vi "题目2.vi"() -> ()   [LabVIEW 2017]
uses:
  <vilib>/Waveform/WDTFileIO.llb/ Write Waveform to File.vi
  <vilib>/Waveform/WDTFileIO.llb/Read Waveform from File.vi
  <vilib>/measure/NI_MABase.lvlib
panel:
  out "first waveform in record":waveform(dbl) caption="记录中第一波形"
  out "波形图":waveform(dbl)(graph)
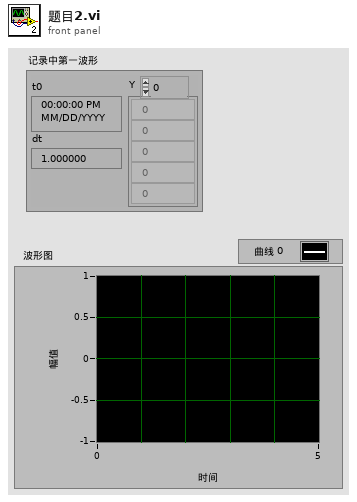
[diagram p1: front panel]
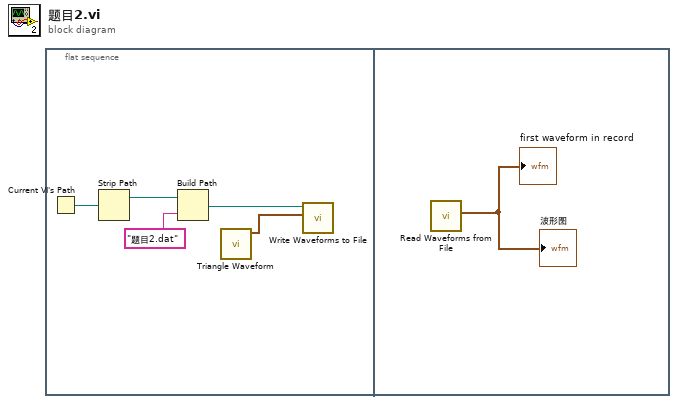
[diagram p0: block diagram]
diagram:
  n1 = flat-sequence {
    frame #0 {
      n2 = Current VI's Path() -> (path=w5:path)
      n3 = Strip Path(path=w5) -> (stripped path=w4:path)  [unwired: 1 out]
      n4 = Build Path(base path=w4, name or relative path="题目2.dat") -> (appended path=w2:path)
      n5 = call <vilib>:"Triangle Waveform.vi"() -> ("signal out"=w1:waveform(dbl))  [unwired: 10 in, 1 out]
      n6 = call-poly <vilib>:"Write Waveforms to File.vi"("waveform"=w1, "file path (dialog if empty)"=w2) -> ()  [unwired: 8 in, 2 out]
    }
    frame #1 {
      n7 = call-poly <vilib>:"Read Waveforms from File.vi"() -> ("first waveform in record"=→"波形图" →"first waveform in record":waveform(dbl))  [unwired: 6 in, 3 out]
    }
  }
